vi "ge_GreyOutCell.vi"(5 "V Ranges":u16[](array[numeric])) -> (2 "Color":u32)   [LabVIEW 2018]
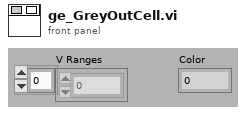
[diagram p1: front panel]
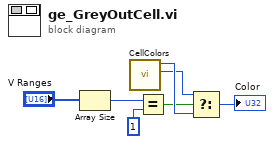
[diagram p0: block diagram]
diagram:
  n1 = Array Size(array="V Ranges") -> (size(s)=w2:i32)
  n2 = call "CellColors.vi"() -> ("Disabled"=w6:u32, "Normal"=w7:u32)  [unwired: 8 in, 2 out]
  n3 = Equal?(x=w2, y=1 ("index")) -> (x = y?=w4:bool)
  n4 = Select(t=w6, s=w4, f=w7) -> (s? t:f=→"Color":u32)
